vi "Prompt for Switches JSON Path.vi"(8 "error in (no error)":errorcluster) -> (0 "error out":errorcluster, 2 "ok?":bool, 3 "selected path":path)   [LabVIEW 2020, in "SLSC Switch System Explorer.lvlib"]
uses:
  SLSC Switch System Explorer.lvlib
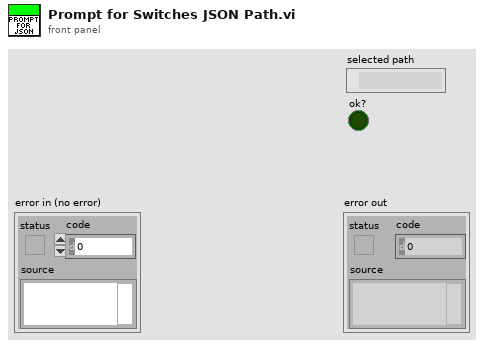
[diagram p1: front panel]
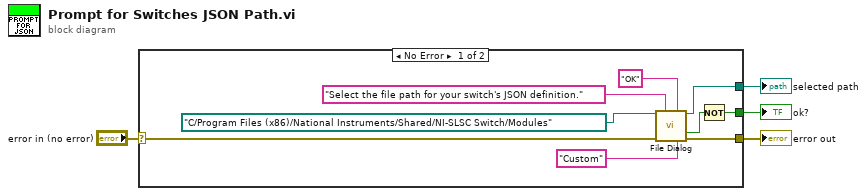
[diagram p0: block diagram]
diagram:
  n1 = case shown="No Error" "error in (no error)" {
    selector: "error in (no error)" -> [w10 w14]
    tunnel: [w9 w14] -> w4
    tunnel: [w8 _] -> w2
    tunnel: [w6 _] -> w1
    frame No Error {
      n2 = call "File Dialog"("start path"=path "C:/Program Files (x86)/National Instruments/Shared/NI-SLSC Switch/Modules", "prompt"="Select the file path for your switch's JSON definition.", "button label"="OK", "error in"=w10, "pattern label"="Custom") -> ("selected path"=w8:path, "cancelled"=w7:bool, "error out"=w9:errorcluster)  [unwired: 7 in, 1 out]
      n3 = Not(x=w7) -> (.not. x?=w6:bool)
    }
    frame Error {
    }
  }
  "error out" <- w4
  "selected path" <- w2
  "ok?" <- w1
